vi "SET Mouse State.vi"(8 "Error In":errorcluster, 11 "Mouse State In":T1) -> (0 "Error Out":errorcluster)   [LabVIEW 2014]
uses:
  Controls/GMap Mouse States.ctl
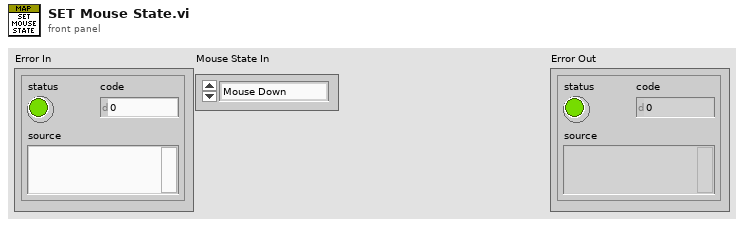
[diagram p1: front panel]
types:
  T1 = typedef "GMap Mouse States.ctl" = enum16{"Mouse Down", "Mouse Up"}
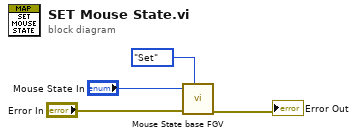
[diagram p0: block diagram]
diagram:
  n1 = call "Mouse State base FGV .vi"("Method"=enum16{"Get", "Set"}."Set", "Error In"="Error In", "Mouse State In"="Mouse State In") -> ("Error Out"=→"Error Out":errorcluster)  [unwired: 7 in, 1 out]
